vi "Ping Dispatcher.vi"(0 "receiver host (\"\")":string, 5 "receiver port (0)":u16, 9 "timeout (100 ms)":i32=100, 11 "error in":errorcluster) -> (4 "response message":T1, 6 "string response":string, 15 "error out":errorcluster)   [LabVIEW 2014, in "AMC.lvlib"]
doc: "Pings the Dispatcher in the application instance specified by \"receiver host\" and \"receiver port\".\n\nIf \"receiver port\" is undefined, this VI will attempt to use the default UDP port."
uses:
  AMC.lvlib
  Message.ctl
  <vilib>/NI/Tools/Keyed Array/KeyedArray.ctl
  <vilib>/NI/Tools/Keyed Array/Map String.vi
  <vilib>/NI/Tools/String/Get Case Matching.vi
  Globals.vi
  <vilib>/NI/Tools/Keyed Array/Tools_KeyedArray.lvlib
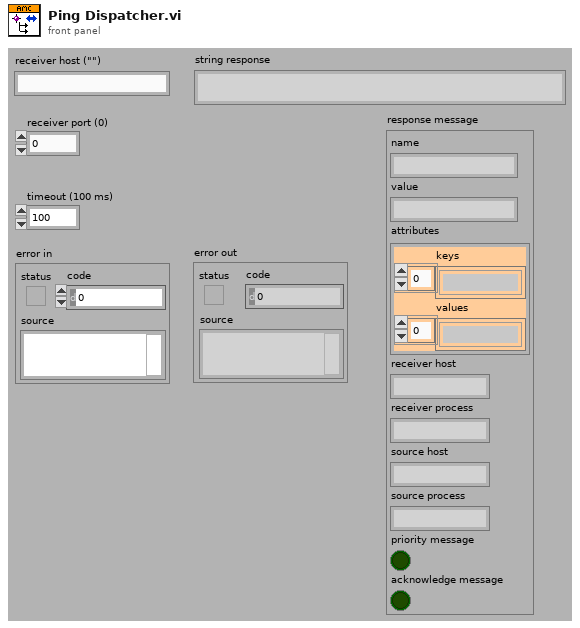
[diagram p1: front panel]
types:
  T1 = typedef "AMC.lvlib/Message.ctl" = cluster{"name":string, "value":string, "attributes":T2, "receiver host":string, "receiver process":string, "source host":string, "source process":string, "priority message":bool, "acknowledge message":bool}
  T2 = typedef "Tools_KeyedArray.lvlib/KeyedArray.ctl" = cluster{"keys":string[], "values":string[]}
  T3 = typedef "AMC.lvlib/Message Queue.ctl" = refnum<queue>
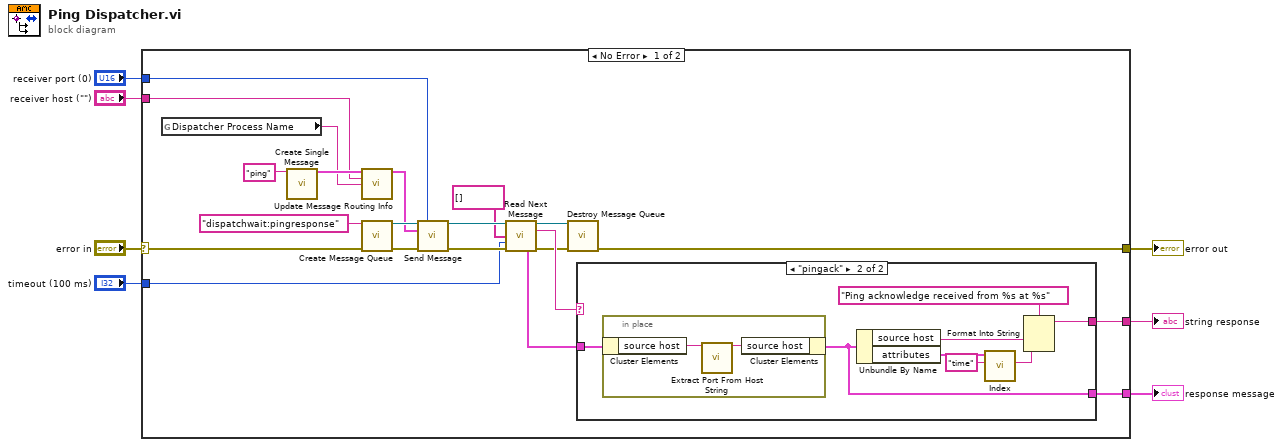
[diagram p0: block diagram]
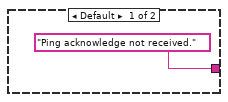
[diagram p2: hidden frame]
diagram:
  n1 = case shown="No Error" "error in" {
    selector: "error in" -> [w17 w40]
    tunnel: [w28 _] -> w7
    tunnel: [w27 _] -> w6
    tunnel: [w26 w40] -> w5
    tunnel: "timeout (100 ms)" -> [w9 _]
    tunnel: "receiver host (\"\")" -> [w14 _]
    tunnel: "receiver port (0)" -> [w10 _]
    frame No Error {
      n2 = global read "Globals.vi" "Dispatcher Process Name"() -> (w13:string)
      n3 = call "Create Single Message.vi"("name"="ping") -> ("message"=w16:T1)  [unwired: 13 in, 1 out]
      n4 = call "Update Message Routing Info.vi"("message"=w16, "receiver host (\"\")"=w14, "receiver process (\"\")"=w13) -> ("message"=w15:T1)  [unwired: 11 in, 1 out]
      n5 = call "Create Message Queue.vi"("message queue name"="dispatchwait:pingresponse", "error in"=w17) -> ("message queue out"=w21:T3, "error out"=w24:errorcluster)  [unwired: 12 in]
      n6 = call "Send Message.vi"("message queue in"=w21, "receiver port"=w10, "message"=w15, "error in"=w24) -> ("message queue out"=w20:T3, "error out"=w25:errorcluster)  [unwired: 9 in, 1 out]
      n7 = call "Read Next Message.vi"("message queue in"=w20, "termination list ([Exit])"=string[] [], "timeout (1 ms)"=w9, "error in"=w25) -> ("message queue out"=w11:T3, "message name"=w19:string, "message"=w18:T1, "error out"=w12:errorcluster)  [unwired: 4 in, 4 out]
      n8 = call "Destroy Message Queue.vi"("message queue in"=w11, "error in"=w12) -> ("error out"=w26:errorcluster)  [unwired: 11 in, 2 out]
      n9 = case shown="\"pingack\"" w19 {
        tunnel: w18 -> [_ w31]
        tunnel: ["Ping acknowledge not received." w32] -> w28
        tunnel: [_ w30] -> w27
        frame Default {
        }
        frame "pingack" {
          n10 = in-place {
            n11 = in-place-cluster #1(w31) -> ("source host"=w39:string)
            n12 = call "Extract Port From Host String.vi"("host in"=w39) -> ("host out"=w38:string)  [unwired: 12 in, 2 out]
            n13 = in-place-cluster #1("source host"=w38) -> (w30:T1)
          }
          n14 = Unbundle By Name(w30) -> ("source host"=w37:string, "attributes"=w34:T2)
          n15 = call <vilib>:"Index.vi"("key"="time", "array in"=w34) -> ("value"=w36:string)  [unwired: 2 in, 3 out]
          n16 = Format Into String(format string="Ping acknowledge received from %s at %s", w37, w36) -> (resulting string=w32:string)  [unwired: 2 in, 1 out]
        }
      }
    }
    frame Error {
    }
  }
  "error out" <- w5
  "string response" <- w7
  "response message" <- w6
